vi "ProcessSeveral.vi"() -> ()   [LabVIEW 2018]
uses:
  MainFGV/Settings/Advanced/AdvancedConfig.ctl
  results_data.ctl
  GraphMean/plot_props.ctl
  GraphMean/axis_props.ctl
  <vilib>/Heliosphere Research LLC/Advanced Plotting Toolkit/api_core/NewPlotScales.ctl
  GraphMean/data_mean_plot.ctl
  <vilib>/Analysis/NI_AALPro.lvlib
  <vilib>/Heliosphere Research LLC/Advanced Plotting Toolkit/Advanced Plotting Toolkit.lvlib
panel:
  in  "PicsDir":path=path "C:/Users/l01481/Desktop/nada" caption="Diretório das imagens"
  in  "stop":bool
  in  "log":bool
  in  "alpha":dbl=0.3 caption="Alpha" format="%#_6f"
  in  "maxFreq":dbl=72.0 caption="Frequência máxima" format="%#_g Hz"
  in  "minFreq":dbl=30.0 caption="Frequência mínima" format="%#_g Hz"
  in  "lowPass":dbl=1000.0 caption="Passa baixa" format="%#_g Hz"
  in  "highPass":dbl=1.0 caption="Passa alta" format="%#_g Hz"
  in  "Filtro":T1(ring)=enum."Passa banda"
  in  "cutoff":dbl=-6.0 caption="Cutoff amplitude [dB]" format="%#_g dB"
  in  "delete":bool
  in  "ok":bool
  in  "validate":bool
  in  "tab":enum32{"Batida individual", "Resultados médios"}(tab)
  out "inert":waveform(dbl)[](graph) caption="Inertância"
  out "hammerSpec":waveform(dbl)(graph) caption="Martelo - Espectro"
  out "acelTime":waveform(dbl)[](graph) caption="Acelerômetros - Sinal no tempo"
  out "hammerTime":waveform(dbl)(graph) caption="Martelo - Sinal no tempo"
  out "meanInert":picture
  in  "TestDir":path=path "C:/Users/l01481/Desktop/nada" caption="Diretório do ensaio"
  # "Análise modal\n\nAquisição\n\nLink do repositório: https://github.com/LeonardoSirino/ModalAnalysis"
  # "Configurações para\napresentação"
  # "Leonardo Sirino\nSistemas Mecânicos \nT + 55 (41) 3361-6152 | C + 55 (41) 99679-007\nleonardo.sirino@lactec.org.br | www.lactec.org.br"
  # "Configurações para\nprocessamento"
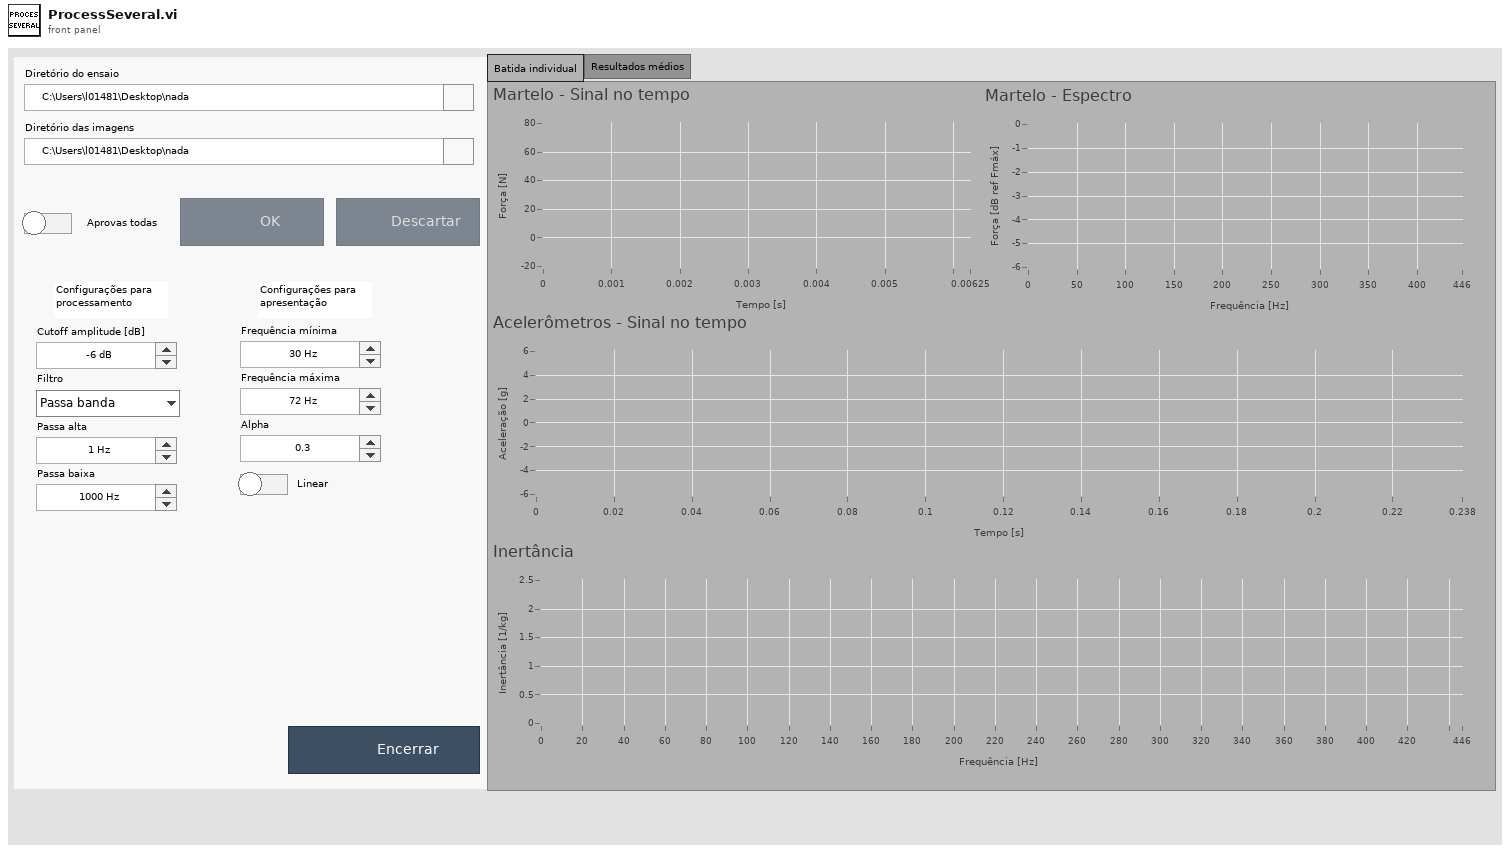
[diagram p1: front panel]
types:
  T1 = enum16{"Desativado", "Passa banda", "Passa alta", "Passa baixa"}
  T2 = typedef "AdvancedConfig.ctl" = cluster{"rate":dbl, "duration":dbl, "thr":dbl, "preTrigger":dbl, "cutoff":dbl, "Filtro":enum16{"Desativado", "Passa banda", "Passa alta", "Passa baixa"}, "highPass":dbl, "lowPass":dbl, "updateTime":dbl}
  T3 = typedef "Advanced Plotting Toolkit.lvlib/NewPlotScales.ctl" = enum16{"Default", "Linear", "Log", "Symlog"}
  T4 = typedef "plot_props.ctl" = cluster{"x_axis":T5, "y_axis":T5, "y multiplier":dbl, "alpha":dbl, "base_tag":string, "itens_base_name":string, "graph_title":string, "plot_names":string[], "plot_all":bool}
  T5 = typedef "axis_props.ctl" = cluster{"min":dbl, "max":dbl, "label":string, "scale":T3}
  T6 = typedef "results_data.ctl" = cluster{"config":T2, "hammer":waveform(dbl), "acelerometers":waveform(dbl)[], "hammerIndex":i32}
  T7 = cluster{"seconds since 1Jan1904":timestamp, "data_out":T6}
  T8 = typedef "data_mean_plot.ctl" = cluster{"array":dbl[], "dx":dbl, "x0":dbl}
  T9 = enum8{"Enabled", "Disabled", "Disabled and Grayed Out"}
  T10 = cluster{"seconds since 1Jan1904":timestamp, "data_out":T6}[]
  T11 = typedef "imagedata.ctl" = cluster{"image type":i32, "image depth":i32, "image":u8[], "mask":u8[], "colors":u32[], "Rectangle":cluster{"left":i16, "top":i16, "right":i16, "bottom":i16}}
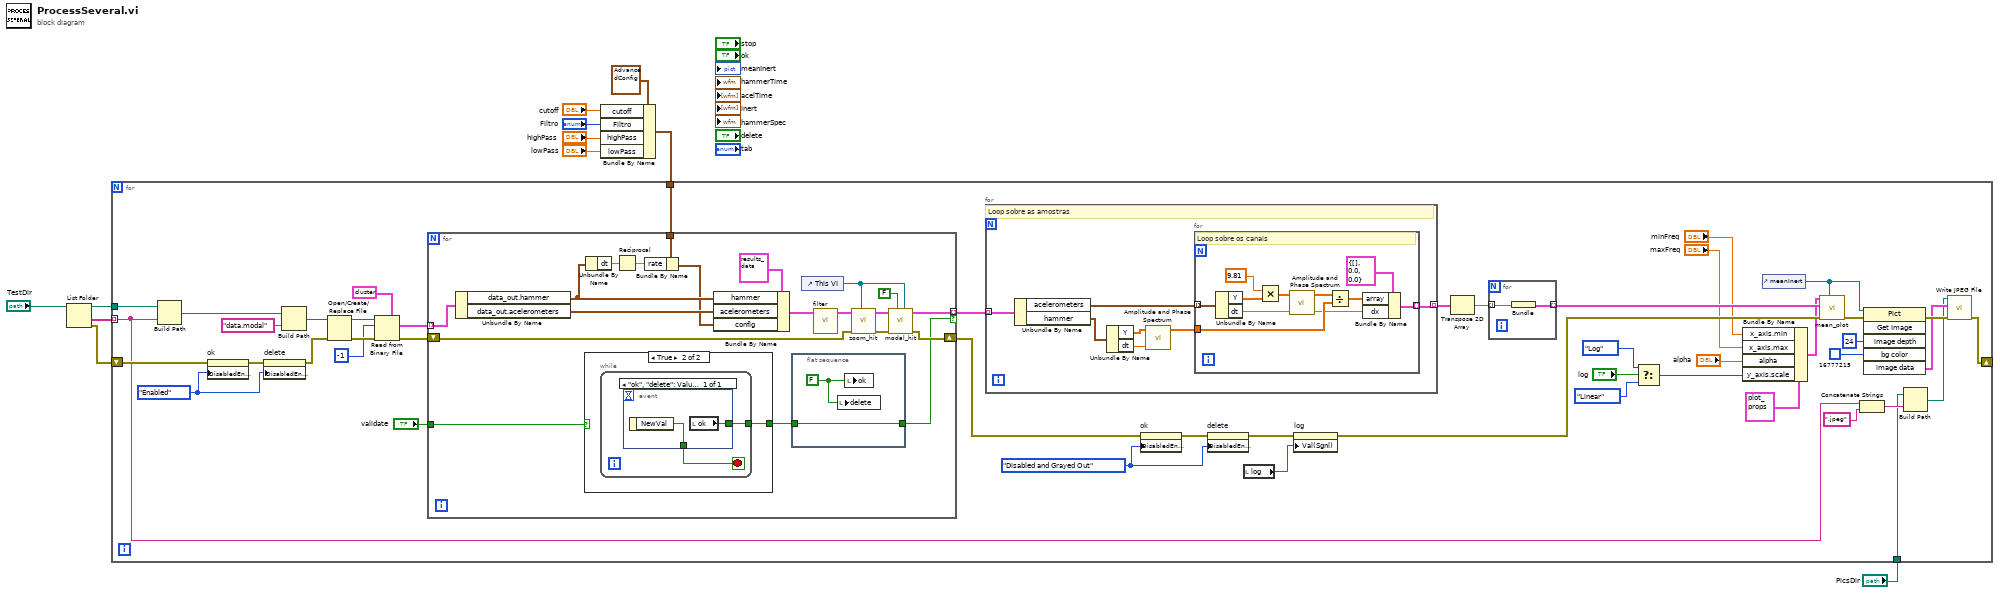
[diagram p0: block diagram]
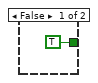
[diagram p2: hidden frame]
diagram:
  n1 = List Folder(path="TestDir") -> (path out=w4:path, folder names=w3:string[], error out=w2:errorcluster)  [unwired: 3 in, 1 out]
  n2 = Bundle By Name(cluster=T2 {"rate"=1652.0, "duration"=1.0, "thr"=10.0, "preTrigger"=100.0, "cutoff"=-6.0, "Filtro"=enum."Passa banda", "highPass"=1.0, "lowPass"=1000.0, "updateTime"=50.0} ("config"), "cutoff"="cutoff", "Filtro"="Filtro", "highPass"="highPass", "lowPass"="lowPass") -> (w6:T2)
  n3 = for {
    tunnel: w6 -> [w51]
    tunnel: w4 -> [w26]
    tunnel: w3 -> [w17] mode=indexing
    shift-right: [w12] -> _
    shift-left: w2 -> [w25]
    tunnel: "PicsDir" -> [w14]
    w38 = T9."Enabled" ("Disabled")
    w40 = T9."Disabled and Grayed Out" ("Disabled")
    n4 = Build Path(base path=w26, name or relative path=w17) -> (appended path=w24:path)
    n5 = property on="ok" class="Bool (strict)"(error in=w25, "DisabledEnum"=w38) -> (error out=w37:errorcluster)  [unwired: 1 in, 1 out]
    n6 = property on="delete" class="Bool (strict)"(error in=w37, "DisabledEnum"=w38) -> (error out=w36:errorcluster)  [unwired: 1 in, 1 out]
    n7 = Build Path(base path=w24, name or relative path="data.modal") -> (appended path=w57:path)
    n8 = Open/Create/Replace File(file path (use dialog)=w57, error in=w36) -> (refnum out=w56:refnum<file>, error out=w54:errorcluster)  [unwired: 4 in, 1 out]
    n9 = Read from Binary File(5:T7 {"seconds since 1Jan1904"=timestamp(0 s since 1904-01-01), "data_out"={"config"={"rate"=0.0, "duration"=0.0, "thr"=0.0, "preTrigger"=0.0, "cutoff"=0.0, "Filtro"=enum."Desativado", "highPass"=0.0, "lowPass"=0.0, "updateTime"=0.0}, "hammer"={"t0"=timestamp(0 s since 1904-01-01), "dt"=1.0, "Y"=[]}, "acelerometers"=[], "hammerIndex"=0}} ("output cluster"), 8:w54, 10:-1 ("count (1)"), 11:w56) -> (0:w50:errorcluster, 2:w52:T10)  [unwired: 2 in, 2 out]
    n10 = for {
      tunnel: w52 -> [w98] mode=indexing
      tunnel: w51 -> [w88]
      shift-right: [w83] -> w42
      shift-left: w50 -> [w84]
      tunnel: [w81] -> w48 mode=indexing if=w80
      tunnel: "validate" -> [w79]
      n11 = Unbundle By Name(w98) -> ("data_out.hammer"=w89:waveform(dbl), "data_out.acelerometers"=w93:waveform(dbl)[])
      n12 = case shown="True" w79 {
        tunnel: [TRUE ("ok") w102] -> w82
        frame False {
        }
        frame True {
          n13 = while {
            tunnel: [w104] -> w102
            stop <- w103 stop-if-true
            n14 = event shown="[0] \"ok\", \"delete\": Value Change" {
              selector: _ -> [_]
              dyn-events: _ -> [_]
              timeout: _ -> [_]
              tunnel: [w105] -> w104
              tunnel: [w106] -> w103
              event "ok", "delete": Value Change {
                n15 = event-data() -> ("NewVal"=w106:bool)  [unwired: 1 in]
                n16 = local read "ok"() -> (w105:bool)
              }
            }
          }
        }
      }
      n17 = Unbundle By Name(w89) -> ("dt"=w87:dbl)
      n18 = Reciprocal(x=w87) -> (1/x=w86:dbl)
      n19 = Bundle By Name(cluster=w88, "rate"=w86) -> (w85:T2)
      n20 = Bundle By Name(cluster=T6 {"config"={"rate"=0.0, "duration"=0.0, "thr"=0.0, "preTrigger"=0.0, "cutoff"=0.0, "Filtro"=enum."Desativado", "highPass"=0.0, "lowPass"=0.0, "updateTime"=0.0}, "hammer"={"t0"=timestamp(0 s since 1904-01-01), "dt"=1.0, "Y"=[]}, "acelerometers"=[], "hammerIndex"=0} ("data_in"), "hammer"=w89, "acelerometers"=w93, "config"=w85) -> (w92:T6)
      n21 = flat-sequence {
        tunnel: w82 -> [w100]
        tunnel: [w100] -> w80
        frame #0 {
          w99 = FALSE ("ok")
          n22 = local write "delete"(w99) -> ()
          n23 = local write "ok"(w99) -> ()
        }
      }
      n24 = control-ref of="This VI"() -> (w91:refnum<vi>)
      n25 = call "filter.vi"("data_in"=w92) -> ("data_out"=w95:T6)  [unwired: 9 in, 1 out]
      n26 = call "zoom_hit.vi"("refVI"=w91, "error in"=w84, "data_in"=w95) -> ("error out"=w96:errorcluster, "data_out"=w97:T6)  [unwired: 7 in]
      n27 = call "modal_hit.vi"("refVI"=w91, "acquisition"=FALSE, "error in"=w96, "data_in"=w97) -> ("error out"=w83:errorcluster, "data_out"=w81:T6)  [unwired: 6 in]
    }
    n28 = for {
      tunnel: w48 -> [w67] mode=indexing
      tunnel: [w61] -> w47 mode=indexing
      # "Loop sobre as amostras"
      n29 = Unbundle By Name(w67) -> ("acelerometers"=w66:waveform(dbl)[], "hammer"=w63:waveform(dbl))
      n30 = Unbundle By Name(w63) -> ("Y"=w64:dbl[], "dt"=w65:dbl)
      n31 = call <vilib>:"Amplitude and Phase Spectrum.vi"("dt"=w65, "Signal (V)"=w64) -> ("Amp Spectrum Mag (Vrms)"=w62:dbl[])  [unwired: 1 in, 2 out]
      n32 = for {
        tunnel: w66 -> [w78] mode=indexing
        tunnel: w62 -> [w72]
        tunnel: [w68] -> w61 mode=indexing
        # "Loop sobre os canais"
        n33 = Unbundle By Name(w78) -> ("Y"=w77:dbl[], "dt"=w74:dbl)
        n34 = Multiply(x=9.81, y=w77) -> (x*y=w75:dbl[])
        n35 = call <vilib>:"Amplitude and Phase Spectrum.vi"("dt"=w74, "Signal (V)"=w75) -> ("df"=w69:dbl, "Amp Spectrum Mag (Vrms)"=w73:dbl[])  [unwired: 1 in, 1 out]
        n36 = Divide(x=w73, y=w72) -> (x/y=w70:dbl[])
        n37 = Bundle By Name(cluster=T8 {"array"=[], "dx"=0.0, "x0"=0.0} ("data_mean_plot"), "array"=w70, "dx"=w69) -> (w68:T8)
      }
    }
    n38 = property on="ok" class="Bool (strict)"(error in=w42, "DisabledEnum"=w40) -> (error out=w41:errorcluster)  [unwired: 1 in, 1 out]
    n39 = property on="delete" class="Bool (strict)"(error in=w41, "DisabledEnum"=w40) -> (error out=w39:errorcluster)  [unwired: 1 in, 1 out]
    n40 = local read "log"() -> (w45:bool)
    n41 = property on="log" class="Bool (strict)"(error in=w39, "Val(Sgnl)"=w45) -> (error out=w44:errorcluster)  [unwired: 1 in, 1 out]
    n42 = Transpose 2D Array(2D array=w47) -> (transposed array=w46:T8[][])
    n43 = for {
      tunnel: w46 -> [w60] mode=indexing
      tunnel: [w59] -> w43 mode=indexing
      n44 = Bundle(w60) -> (w59:cluster{T8[]})  [unwired: 1 in]
    }
    n45 = Select(t=NewPlotScales."Log" ("y_axis.scale"), s="log", f=NewPlotScales."Linear" ("y_axis.scale")) -> (s? t:f=w35:T3)
    n46 = Bundle By Name(cluster=T4 {"x_axis"={"min"=30.0, "max"=72.0, "label"="Frequência [Hz]", "scale"=enum."Default"}, "y_axis"={"min"=nan, "max"=nan, "label"="Inertância [1/kg]", "scale"=enum."Linear"}, "y multiplier"=1.0, "alpha"=0.5, "base_tag"="", "itens_base_name"="", "graph_title"="Inertância média", "plot_names"=[], "plot_all"=TRUE} ("plot_properties"), "x_axis.min"="minFreq", "x_axis.max"="maxFreq", "alpha"="alpha", "y_axis.scale"=w35) -> (w29:T4)
    n47 = control-ref of="meanInert"() -> (w23:refnum<vi>)
    n48 = call "mean_plot.vi"("ref_picture"=w23, "error in"=w44, "channels"=w43, "plot_properties"=w29) -> ("error out"=w22:errorcluster)  [unwired: 5 in, 2 out]
    n49 = Concatenate Strings(w17, ".jpeg" ("string")) -> (w15:string)
    n50 = invoke class="Pict" method="Get Image"(reference=w23, error in=w22, "image depth"=24 ("Image Depth"), "bg color"=u32 16777215) -> (error out=w21:errorcluster, "image data"=w20:T11)  [unwired: 2 in, 4 out]
    n51 = Build Path(base path=w14, name or relative path=w15) -> (appended path=w13:path)
    n52 = call <vilib>:"Write JPEG File.vi"("error in (no error)"=w21, "image data"=w20, "path to JPEG file"=w13) -> ("error out"=w12:errorcluster)  [unwired: 7 in, 1 out]
  }
